vi "Destroy.vi"(8 "error in (no error)":errorcluster, 11 "Uint32 in":refnum<class "Uint32.lvclass">) -> (0 "error out":errorcluster)   [LabVIEW 2013, in "MDSplus.lvlib" / "Uint32.lvclass"]
uses:
  <vilib>/MDSplus/Classes/Data_Class/Scalar_Class/Uint32_Class/Uint32.lvclass
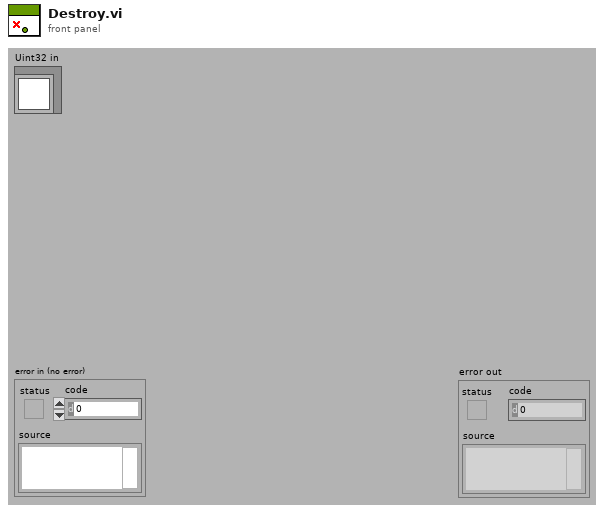
[diagram p1: front panel]
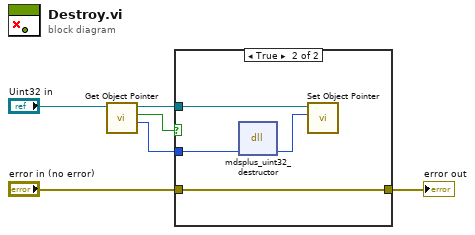
[diagram p0: block diagram]
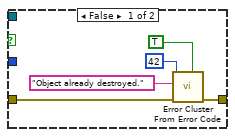
[diagram p2: hidden frame]
diagram:
  n1 = call-dynamic "Get Object Pointer.vi"("Data in"="Uint32 in") -> ("Object Pointer"=w4:i64, "Assigned object pointer?"=w5:bool, "Data out"=w6:refnum<class "Uint32.lvclass">)  [unwired: 8 in]
  n2 = case shown="True" w5 {
    tunnel: w6 -> [_ w15]
    tunnel: w4 -> [_ w14]
    tunnel: "error in (no error)" -> [w11 w12]
    tunnel: [w8 w12] -> w1
    frame False {
      n3 = call <vilib>:"Error Cluster From Error Code.vi"("is warning? (False)"=TRUE, "error in (no error)"=w11, "error message (\"\")"="Object already destroyed." ("error message (\"\")"), "error code (0)"=42) -> ("error out"=w8:errorcluster)  [unwired: 5 in]
    }
    frame True {
      n4 = dll-call lib="MDSobjectsLVShr" fn="mdsplus_uint32_destructor"("lvUint32Ptr"=w14) -> ("lvUint32Ptr"=w13:i64)  [unwired: 4 in, 2 out]
      n5 = call-dynamic "Set Object Pointer.vi"("Object Pointer"=w13, "Data in"=w15) -> ()  [unwired: 9 in, 1 out]
    }
  }
  "error out" <- w1
